vi "IonGauge.vi"(3 "Index":i32[](array[numeric]), 4 "Voltage":u32[](array[numeric]), 5 "Scale":dbl[](array[numeric]) format="%.2f") -> (1 "Scale out":dbl[](array[numeric]) format="%.2f")   [LabVIEW 2011]
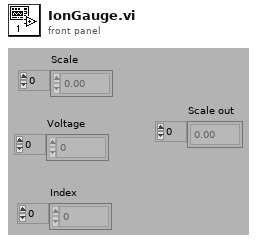
[diagram p1: front panel]
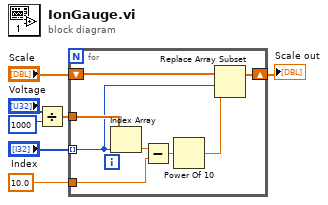
[diagram p0: block diagram]
diagram:
  n1 = Divide(x="Voltage", y=1000) -> (x/y=w4:dbl[])
  n2 = for {
    tunnel: "Index" -> [w10] mode=indexing
    tunnel: w4 -> [w15]
    tunnel: 10.0 -> [w12]
    shift-right: [w9] -> w1
    shift-left: "Scale" -> [w11]
    n3 = Index Array(array=w15, index=w10) -> (element=w14:dbl)
    n4 = Subtract(x=w14, y=w12) -> (x-y=w13:dbl)
    n5 = Power Of 10(x=w13) -> (10^x=w8:dbl)
    n6 = Replace Array Subset(array=w11, new element=w8, index=w10) -> (w9:dbl[])
  }
  "Scale out" <- w1
